vi "senser.vi"(1 "待处理数据":u8[](array[numeric])) -> (0 "输出簇":T1)   [LabVIEW 2014]
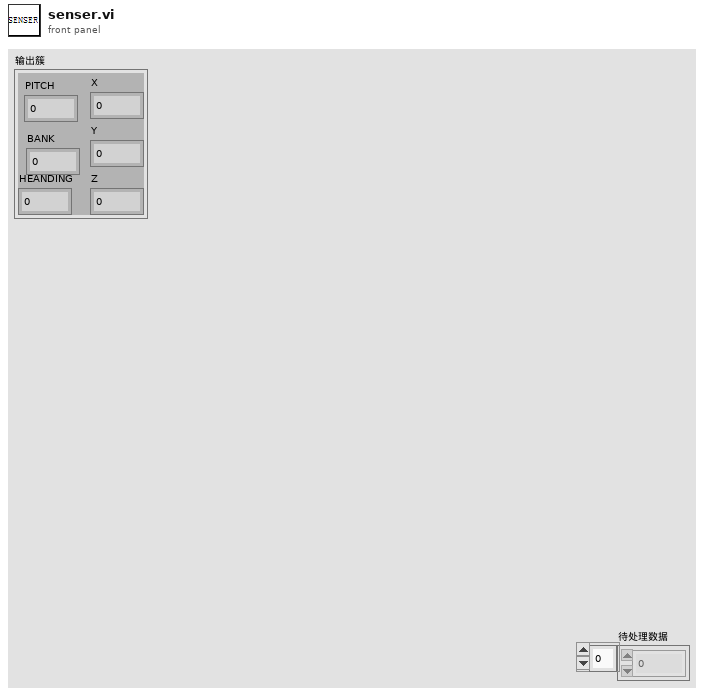
[diagram p1: front panel]
types:
  T1 = cluster{"PITCH":i32, "BANK":i32, "HEANDING":i32, "X":i32, "Y":i32, "Z":i32}
  T2 = cluster{"32位整型":i32, "32位整型":i32, "32位整型":i32, "32位整型":i32, "32位整型":i32, "32位整型":i32}
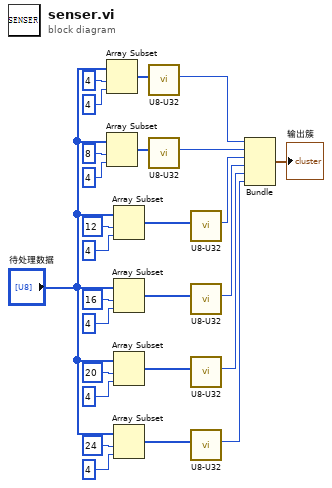
[diagram p0: block diagram]
diagram:
  n1 = Array Subset(array="待处理数据", index=4 ("长度（剩余）"), length=4 ("长度（剩余）")) -> (w17:u8[])
  n2 = Array Subset(array="待处理数据", index=8 ("长度（剩余）"), length=4 ("长度（剩余）")) -> (w14:u8[])
  n3 = Array Subset(array="待处理数据", index=12 ("长度（剩余）"), length=4 ("长度（剩余）")) -> (w4:u8[])
  n4 = Array Subset(array="待处理数据", index=16 ("长度（剩余）"), length=4 ("长度（剩余）")) -> (w3:u8[])
  n5 = Array Subset(array="待处理数据", index=20 ("长度（剩余）"), length=4 ("长度（剩余）")) -> (w2:u8[])
  n6 = Array Subset(array="待处理数据", index=24 ("长度（剩余）"), length=4 ("长度（剩余）")) -> (w1:u8[])
  n7 = call "U8-U32.vi"("数组"=w17) -> ("32位整型"=w25:i32)  [unwired: 8 in, 1 out]
  n8 = call "U8-U32.vi"("数组"=w14) -> ("32位整型"=w24:i32)  [unwired: 8 in, 1 out]
  n9 = call "U8-U32.vi"("数组"=w4) -> ("32位整型"=w23:i32)  [unwired: 8 in, 1 out]
  n10 = call "U8-U32.vi"("数组"=w3) -> ("32位整型"=w20:i32)  [unwired: 8 in, 1 out]
  n11 = call "U8-U32.vi"("数组"=w2) -> ("32位整型"=w22:i32)  [unwired: 8 in, 1 out]
  n12 = call "U8-U32.vi"("数组"=w1) -> ("32位整型"=w21:i32)  [unwired: 8 in, 1 out]
  n13 = Bundle("32位整型"=w25, "32位整型"=w24, "32位整型"=w23, "32位整型"=w20, "32位整型"=w22, "32位整型"=w21) -> (→"输出簇":T2)  [unwired: 1 in]
